vi "protocoll version.vi"() -> ()   [LabVIEW 2018, in "LV-0mq-Julia_roundtrip-lib.lvlib"]
uses:
  LV-0mq-Julia_roundtrip-lib.lvlib
panel:
  out "PROTOC_V":u8=1
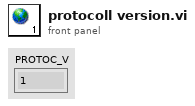
[diagram p1: front panel]
diagram:
